vi "ex_PPGetProp.vi"(0 "Output Cluster":T1, 1 "Suffix":string, 2 "CR/LF":string="\n", 5 "Previous String":string, 7 "Enum & T/F Strings":string[](array[string]), 9 "Prefix":string, 11 "Control:":string) -> (3 "Enum Result":string, 4 "String":string, 6 "int32":i32, 8 "dbl":dbl format="%0.2f", 10 "bool":bool, 12 "String (Path)":string, 13 "Int32 String":string, 14 "T/F Result":string, 15 "dbl String":string)   [LabVIEW 2017]
doc: "Specifies the value of the specified control for many different data types given references to both VIs and their controls, the Control Data array, and the name of the control you are looking for."
uses:
  <vilib>/express/express shared/propPageData.ctl
panel:
  in  "Control not found while generating help.  Property:":string="Control not found while generating help.  Property: "
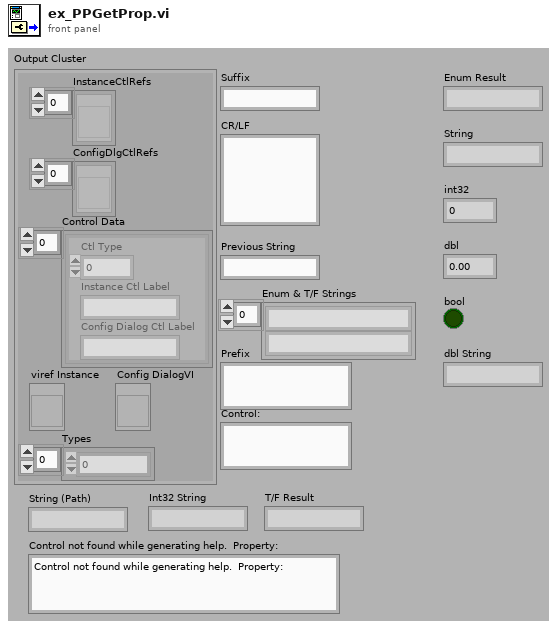
[diagram p1: front panel]
types:
  T1 = typedef "propPageData.ctl" = cluster{"InstanceCtlRefs":refnum<vi>[], "ConfigDlgCtlRefs":refnum<vi>[], "Control Data":cluster{"Ctl Type":u16, "Instance Ctl Label":string, "Config Dialog Ctl Label":string}[], "viref Instance":refnum<vi>, "Types":i32[], "Config DialogVI":refnum<vi>}
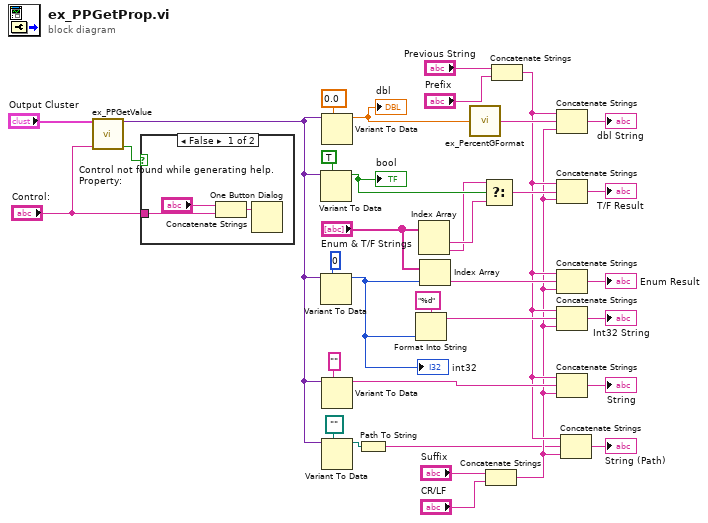
[diagram p0: block diagram]
diagram:
  n1 = call <vilib>:"ex_PPGetValue.vi"("Control Data"="Output Cluster", "Control:"="Control:") -> ("Value"=w10:variant, "Found"=w1:bool)  [unwired: 12 in]
  n2 = case shown="False" w1 {
    tunnel: "Control:" -> [w36 _]
    frame False {
      n3 = Concatenate Strings("Control not found while generating help.  Property:", w36) -> (w37:string)
      n4 = One Button Dialog(message=w37) -> ()  [unwired: 1 in, 1 out]
    }
    frame True {
    }
  }
  n5 = Variant To Data(type=TRUE, Variant=w10) -> (data=w29:bool)  [unwired: 1 in, 1 out]
  "bool" <- w29
  n6 = Variant To Data(type=0, Variant=w10) -> (data=w18:i32)  [unwired: 1 in, 1 out]
  "int32" <- w18
  n7 = Variant To Data(type=0.0, Variant=w10) -> (data=w12:dbl)  [unwired: 1 in, 1 out]
  "dbl" <- w12
  n8 = Variant To Data(type="", Variant=w10) -> (data=w15:string)  [unwired: 1 in, 1 out]
  n9 = Variant To Data(type=path "", Variant=w10) -> (data=w8:path)  [unwired: 1 in, 1 out]
  n10 = Path To String(path=w8) -> (string=w5:string)
  n11 = Format Into String(format string="%d" ("Format String"), w18) -> (resulting string=w17:string)  [unwired: 2 in, 1 out]
  n12 = Index Array(array="Enum & T/F Strings") -> (element #1=w28:string, element #2=w27:string)  [unwired: 2 in]
  n13 = Index Array(array="Enum & T/F Strings", index=w18) -> (element=w24:string)
  n14 = call <vilib>:"ex_PercentGFormat.vi"("Numeric"=w12) -> ("String"=w11:string)  [unwired: 1 in]
  n15 = Select(t=w27, s=w29, f=w28) -> (s? t:f=w31:string)
  n16 = Concatenate Strings("Suffix", "CR/LF") -> (w6:string)
  n17 = Concatenate Strings("Previous String", "Prefix") -> (w7:string)
  n18 = Concatenate Strings(w7, w11, w6) -> (→"dbl String":string)
  n19 = Concatenate Strings(w7, w31, w6) -> (→"T/F Result":string)
  n20 = Concatenate Strings(w7, w24, w6) -> (→"Enum Result":string)
  n21 = Concatenate Strings(w7, w17, w6) -> (→"Int32 String":string)
  n22 = Concatenate Strings(w7, w15, w6) -> (→"String":string)
  n23 = Concatenate Strings(w7, w5, w6) -> (→"String (Path)":string)
